vi "Init Events.vi"(8 "error in (no error)":errorcluster, 11 "HistorianCharting in":refnum<class "HistorianCharting.lvclass">) -> (0 "error out":errorcluster, 3 "HistorianCharting out":refnum<class "HistorianCharting.lvclass">)   [LabVIEW 2020, in "VolatusGUIElements.lvlib" / "HistorianCharting.lvclass"]
uses:
  HistorianCharting.lvclass
  Lock Now Data.ctl
  Plot Color Data.ctl
  Plot Visible Data.ctl
  Scale Data.ctl
  VolatusGUI/Historian Charting Manager/Scale.ctl
  Time Data.ctl
  Events.ctl
  Config Data.ctl
  VolatusGUI/Historian Charting Manager/Select Plot Group Data.ctl
  VolatusGUI/Historian Charting Manager/Plot Group Config.ctl
  VolatusGUI/Historian Charting Manager/X-Axis Type.ctl
  VolatusGUI/Historian Charting Manager/Plot Config.ctl
  HistorianCharting.lvclass/HistorianCharting.ctl
  VolatusGUI/Historian Charting Manager/Historian Charting Manager.lvclass
  Selection Data.ctl
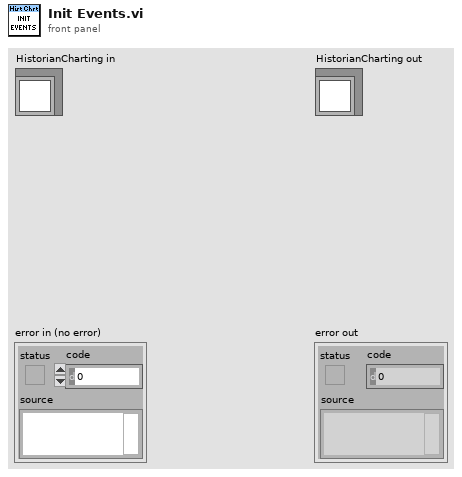
[diagram p1: front panel]
types:
  T1 = typedef "VolatusGUIElements.lvlib/HistorianCharting.lvclass/Selection Data.ctl" = cluster{"Plot Group":string}
  T2 = typedef "VolatusGUI.lvlib/Historian Charting Manager.lvclass/Select Plot Group Data.ctl" = cluster{"Chart Num":i32, "Plots Config":T3}
  T3 = typedef "VolatusGUI.lvlib/Historian Charting Manager.lvclass/Plot Group Config.ctl" = cluster{"Name":string, "X-Axis Type":T4, "X-Axis Channel":string, "Plots":T5[], "Lock Now":bool, "Time":string}
  T4 = typedef "VolatusGUI.lvlib/Historian Charting Manager.lvclass/X-Axis Type.ctl" = enum16{"Time", "Channel"}
  T5 = typedef "VolatusGUI.lvlib/Historian Charting Manager.lvclass/Plot Config.ctl" = cluster{"Channel":string, "Visible":bool, "Color":u32, "Scale":T6}
  T6 = typedef "VolatusGUI.lvlib/Historian Charting Manager.lvclass/Scale.ctl" = enum16{"Left", "Right"}
  T7 = typedef "VolatusGUIElements.lvlib/HistorianCharting.lvclass/Config Data.ctl" = cluster{"Unused":bool}
  T8 = typedef "VolatusGUIElements.lvlib/HistorianCharting.lvclass/Events.ctl" = cluster{"Lock Now":refnum<user-event>, "Plot Color":refnum<user-event>, "Plot Vis":refnum<user-event>, "Scale":refnum<user-event>, "Time":refnum<user-event>, "Config":refnum<user-event>, "Select Plot Group":refnum<user-event>, "Selection":refnum<user-event>}
  T9 = typedef "VolatusGUIElements.lvlib/HistorianCharting.lvclass/Time Data.ctl" = cluster{"New Time":string, "Old Time":string}
  T10 = typedef "VolatusGUIElements.lvlib/HistorianCharting.lvclass/Scale Data.ctl" = cluster{"Index":i32, "Scale":T6}
  T11 = typedef "VolatusGUIElements.lvlib/HistorianCharting.lvclass/Plot Visible Data.ctl" = cluster{"Index":i32, "Visible":bool}
  T12 = typedef "VolatusGUIElements.lvlib/HistorianCharting.lvclass/Plot Color Data.ctl" = cluster{"Index":i32, "Color":u32}
  T13 = typedef "VolatusGUIElements.lvlib/HistorianCharting.lvclass/Lock Now Data.ctl" = cluster{"Lock Now":bool}
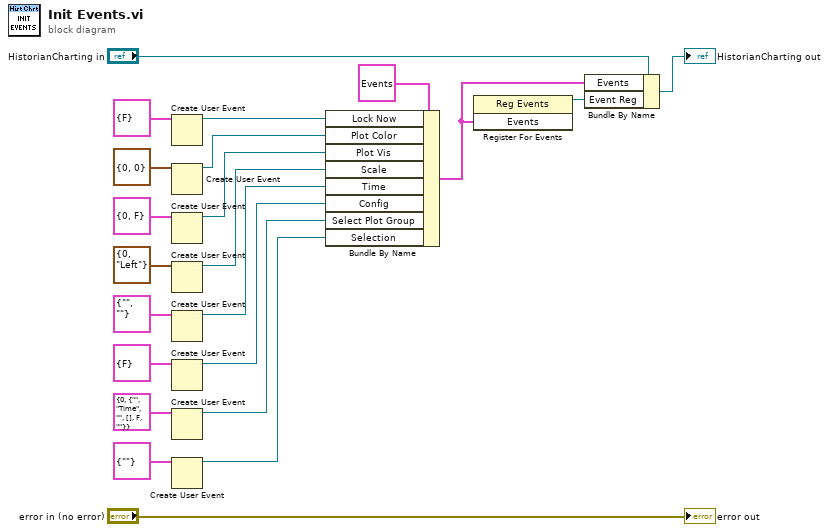
[diagram p0: block diagram]
diagram:
  n1 = Create User Event(user event datatype=T13 {"Lock Now"=FALSE} ("Lock Now Data")) -> (user event=w14:refnum<user-event>)  [unwired: 1 in, 1 out]
  n2 = Create User Event(user event datatype=T12 {"Index"=0, "Color"=0} ("Plot Color Data")) -> (user event=w13:refnum<user-event>)  [unwired: 1 in, 1 out]
  n3 = Create User Event(user event datatype=T11 {"Index"=0, "Visible"=FALSE} ("Plot Visible Data")) -> (user event=w12:refnum<user-event>)  [unwired: 1 in, 1 out]
  n4 = Create User Event(user event datatype=T10 {"Index"=0, "Scale"=enum."Left"} ("Scale Data")) -> (user event=w11:refnum<user-event>)  [unwired: 1 in, 1 out]
  n5 = Create User Event(user event datatype=T9 {"New Time"="", "Old Time"=""} ("Time Data")) -> (user event=w10:refnum<user-event>)  [unwired: 1 in, 1 out]
  n6 = Create User Event(user event datatype=T7 {"Unused"=FALSE} ("Config Data")) -> (user event=w5:refnum<user-event>)  [unwired: 1 in, 1 out]
  n7 = Create User Event(user event datatype=T2 {"Chart Num"=0, "Plots Config"={"Name"="", "X-Axis Type"=enum."Time", "X-Axis Channel"="", "Plots"=[], "Lock Now"=FALSE, "Time"=""}} ("Select Plot Group Data")) -> (user event=w3:refnum<user-event>)  [unwired: 1 in, 1 out]
  n8 = Create User Event(user event datatype=T1 {"Plot Group"=""} ("Selection Data")) -> (user event=w1:refnum<user-event>)  [unwired: 1 in, 1 out]
  n9 = Bundle By Name(cluster=T8 {"Lock Now"=refnum, "Plot Color"=refnum, "Plot Vis"=refnum, "Scale"=refnum, "Time"=refnum, "Config"=refnum, "Select Plot Group"=refnum, "Selection"=refnum} ("Events"), "Lock Now"=w14, "Plot Color"=w13, "Plot Vis"=w12, "Scale"=w11, "Time"=w10, "Config"=w5, "Select Plot Group"=w3, "Selection"=w1) -> (w7:T8)
  n10 = register-events(w7) -> (reference out=w8:refnum<event-registration>)  [unwired: 2 in, 1 out]
  n11 = Bundle By Name(cluster="HistorianCharting in", "Events"=w7, "Event Reg"=w8) -> (→"HistorianCharting out":refnum<class "HistorianCharting.lvclass">)
  "error out" <- "error in (no error)"
